vi "think_and_act.vi"(8 "error in (no error)":errorcluster, 9 "antState":T1, 10 "pieceOfWorld":T4[][](array[typedef]), 11 "Igor_1 in":refnum<class "Igor_1.lvclass">) -> (0 "error out":errorcluster, 2 "action":T2, 3 "Igor_1 out":refnum<class "Igor_1.lvclass">)   [LabVIEW 2015, in "Igor_1.lvclass"]
doc: "Ant thinks and chooses action\nCreated by Artem Shevelev\nshevelev.pro\nartem@shevelev.pro\nLabVIEW Portal: https://labviewportal.org/memberlist.php?mode=viewprofile&u=2340"
uses:
  Igor_1.lvclass
  actors/world/typedefs/worldCell_cluster.ctl
  actors/world/typedefs/markValue_cluster.ctl
  actors/world/typedefs/markValue.ctl
  actors/world/typedefs/markVolume.ctl
  actors/world/typedefs/amountOfFood.ctl
  actors/world/typedefs/anthillType_enum.ctl
  ant_base/action_cluster.ctl
  ant_base/actionType_enum.ctl
  ant_base/antState_cluster.ctl
  ant_base/ant_base.lvclass/ant_base.ctl
  ant_base/memory_limit_const.vi
  ant_base/ant_base.lvclass
  actors/world/world.lvlib
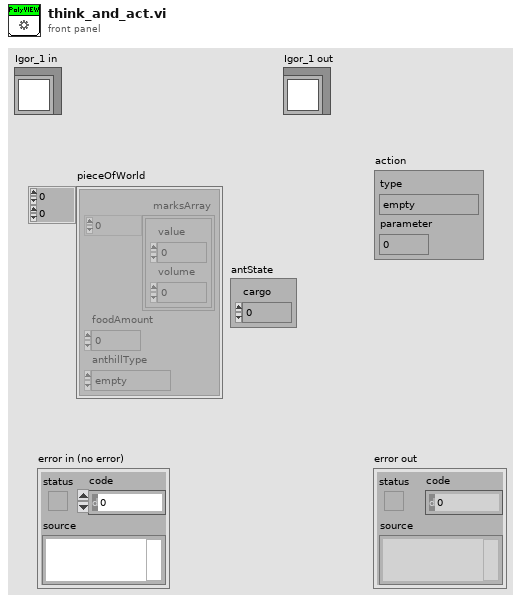
[diagram p1: front panel]
types:
  T1 = typedef "ant_base.lvclass/antState_cluster.ctl" = cluster{"cargo":u8}
  T2 = typedef "ant_base.lvclass/action_cluster.ctl" = cluster{"type":T3, "parameter":dbl}
  T3 = typedef "ant_base.lvclass/actionType_enum.ctl" = enum8{"empty", "move", "take", "put", "mark"}
  T4 = typedef "world.lvlib/worldCell_cluster.ctl" = cluster{"marksArray":T5[], "foodAmount":T8, "anthillType":T9}
  T5 = typedef "world.lvlib/markValue_cluster.ctl" = cluster{"value":T6, "volume":T7}
  T6 = typedef "world.lvlib/markValue.ctl" = u8
  T7 = typedef "world.lvlib/markVolume.ctl" = u16
  T8 = typedef "world.lvlib/amountOfFood.ctl" = i32
  T9 = typedef "world.lvlib/anthillType_enum.ctl" = enum16{"empty", "own", "rival"}
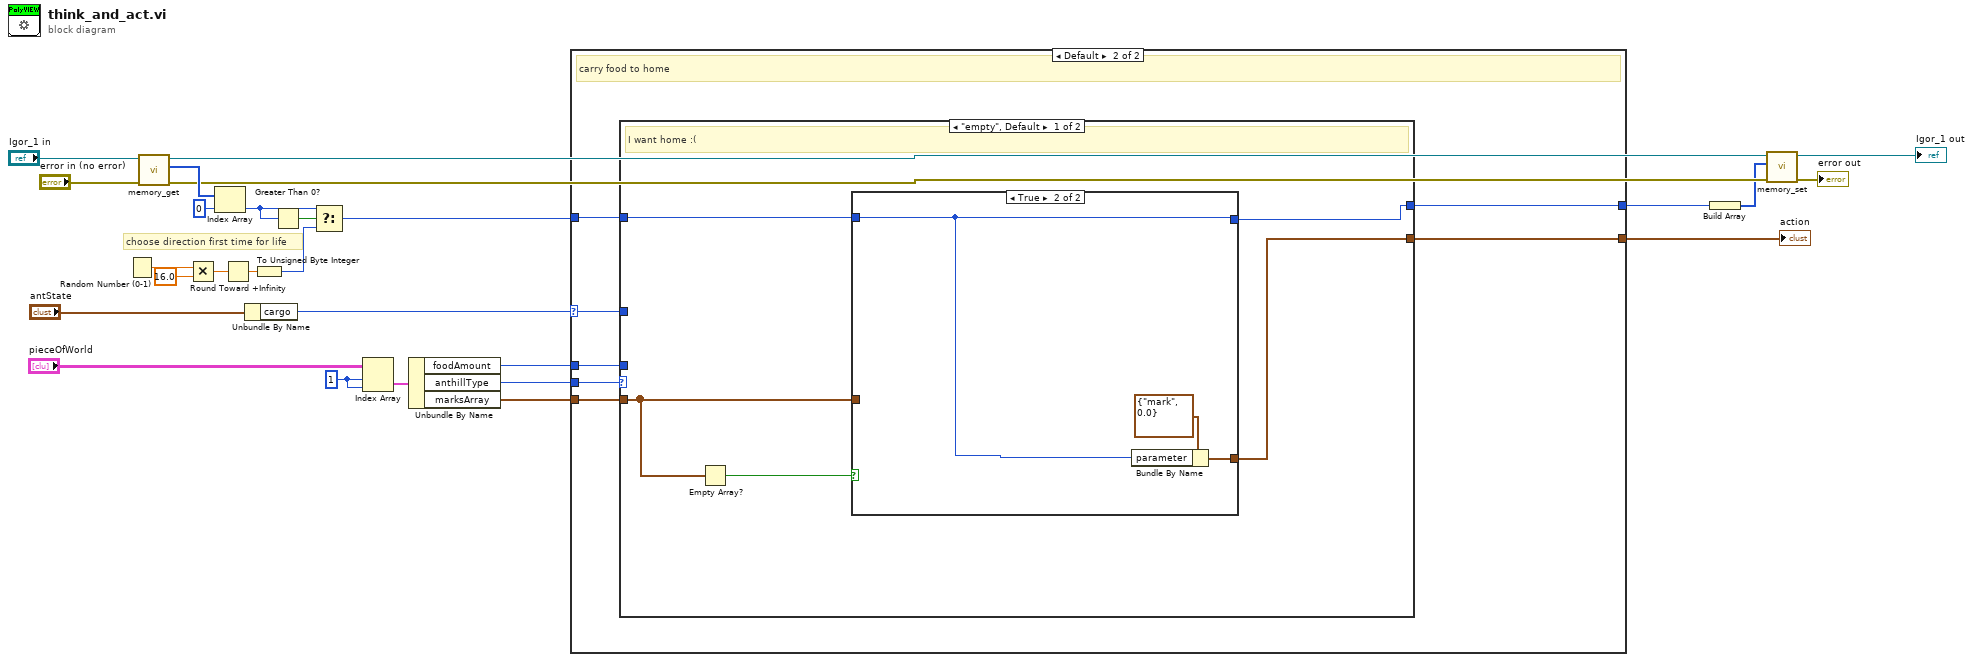
[diagram p0: block diagram]
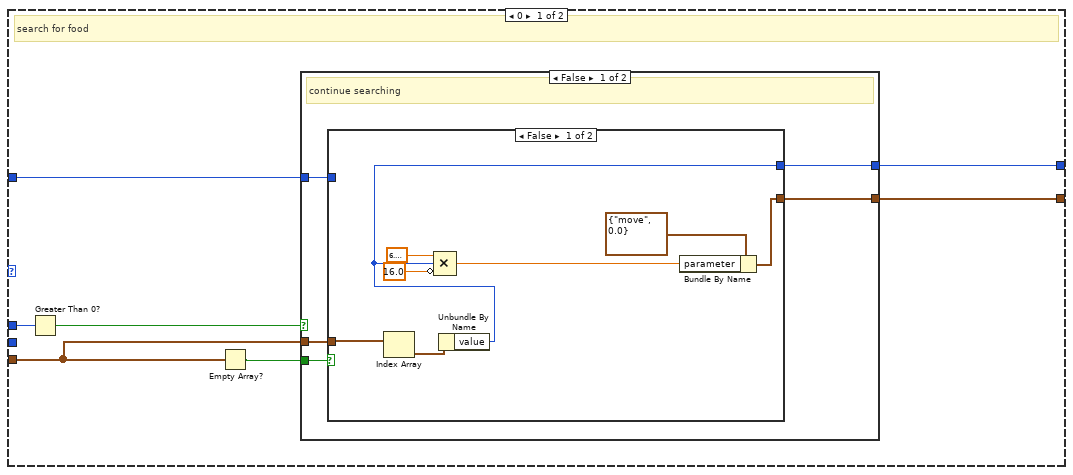
[diagram p2: hidden frame]
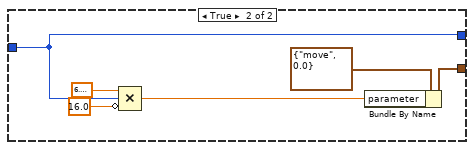
[diagram p3: hidden frame]
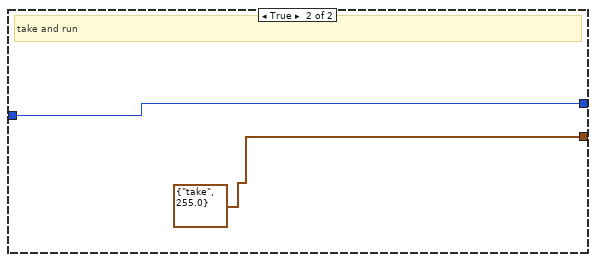
[diagram p4: hidden frame]
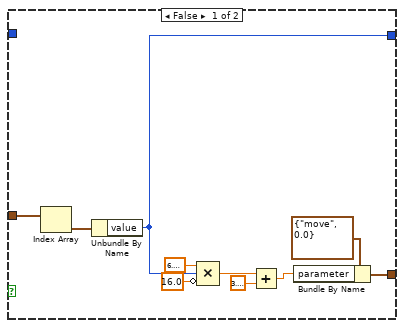
[diagram p5: hidden frame]
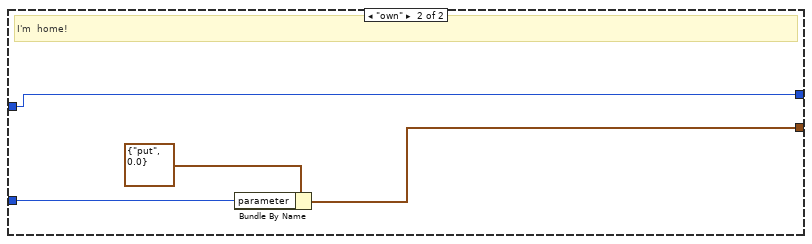
[diagram p6: hidden frame]
diagram:
  w17 = 1 ("index (row)")
  # "choose direction first time for life"
  n1 = Random Number (0-1)() -> (number: 0 to 1=w26:dbl)
  n2 = call "memory_get.vi"("error in (no error)"="error in (no error)", "ant_base in"="Igor_1 in") -> ("error out"=w18:errorcluster, "memory"=w19:u8[], "ant_base out"=w20:refnum<class "Igor_1.lvclass">)  [unwired: 7 in]
  n3 = Multiply(x=w26, y=16.0) -> (x*y=w25:dbl)
  n4 = Index Array(array=w19, index=0) -> (element=w21:u8)
  n5 = Round Toward +Infinity(x=w25) -> (ceil(x): smallest int >= x=w24:dbl)
  n6 = Unbundle By Name("antState") -> ("cargo"=w15:u8)
  n7 = To Unsigned Byte Integer(number=w24) -> (unsigned 8bit integer=w22:u8)
  n8 = Greater Than 0?(x=w21) -> (x > 0?=w23:bool)
  n9 = Select(t=w21, s=w23, f=w22) -> (s? t:f=w7:u8)
  n10 = Index Array(array="pieceOfWorld", index (row)=w17, index (col)=w17) -> (element=w16:T4)
  n11 = Unbundle By Name(w16) -> ("foodAmount"=w14:T8, "anthillType"=w13:T9, "marksArray"=w1:T5[])
  n12 = case shown="Default" w15 {
    selector: w15 -> [_ w59]
    tunnel: w14 -> [w34 w61]
    tunnel: w13 -> [_ w62]
    tunnel: [w32 w60] -> w8
    tunnel: w7 -> [w31 w58]
    tunnel: [w30 w57] -> w6
    tunnel: w1 -> [w28 w56]
    frame 0 {
      # "search for food"
      n13 = Greater Than 0?(x=w34) -> (x > 0?=w33:bool)
      n14 = Empty Array?(array=w28) -> (empty?=w29:bool)
      n15 = case shown="False" w33 {
        tunnel: [w39 T2 {"type"=enum."take", "parameter"=255.0} ("action")] -> w32
        tunnel: w31 -> [w37 w55]
        tunnel: [w38 w55] -> w30
        tunnel: w29 -> [w36 _]
        tunnel: w28 -> [w35 _]
        frame False {
          # "continue searching"
          n16 = case shown="False" w36 {
            tunnel: [w40 w52] -> w39
            tunnel: [w41 w48] -> w38
            tunnel: w37 -> [_ w48]
            tunnel: w35 -> [w47 _]
            frame False {
              n17 = Index Array(array=w47) -> (element=w42:T5)  [unwired: 1 in]
              n18 = Unbundle By Name(w42) -> ("value"=w41:T6)
              n19 = Compound Arithmetic op=MULTIPLY(6.283185307179586, w41, invert 16.0 ("y")) -> (w43:dbl)
              n20 = Bundle By Name(cluster=T2 {"type"=enum."move", "parameter"=0.0} ("action"), "parameter"=w43) -> (w40:T2)
            }
            frame True {
              n21 = Compound Arithmetic op=MULTIPLY(6.283185307179586, w48, invert 16.0 ("y")) -> (w49:dbl)
              n22 = Bundle By Name(cluster=T2 {"type"=enum."move", "parameter"=0.0} ("action"), "parameter"=w49) -> (w52:T2)
            }
          }
        }
        frame True {
          # "take and run"
        }
      }
    }
    frame Default {
      # "carry food to home"
      n23 = case shown="\"empty\", Default" w62 {
        tunnel: w61 -> [_ _]
        tunnel: [w67 w83] -> w60
        tunnel: w59 -> [_ w82]
        tunnel: w58 -> [w65 w81]
        tunnel: [w64 w81] -> w57
        tunnel: w56 -> [w63 _]
        frame "empty", Default {
          # "I want home :("
          n24 = Empty Array?(array=w63) -> (empty?=w66:bool)
          n25 = case shown="True" w66 {
            tunnel: [w76 w79] -> w67
            tunnel: w65 -> [_ w78]
            tunnel: [w68 w78] -> w64
            tunnel: w63 -> [w69 _]
            frame False {
              n26 = Index Array(array=w69) -> (element=w70:T5)  [unwired: 1 in]
              n27 = Unbundle By Name(w70) -> ("value"=w68:T6)
              n28 = Compound Arithmetic op=MULTIPLY(6.283185307179586, w68, invert 16.0 ("y")) -> (w71:dbl)
              n29 = Add(x=w71, y=3.141592653589793) -> (x+y=w75:dbl)
              n30 = Bundle By Name(cluster=T2 {"type"=enum."move", "parameter"=0.0} ("action"), "parameter"=w75) -> (w76:T2)
            }
            frame True {
              n31 = Bundle By Name(cluster=T2 {"type"=enum."mark", "parameter"=0.0} ("action"), "parameter"=w78) -> (w79:T2)
            }
          }
        }
        frame "own" {
          # "I'm  home!"
          n32 = Bundle By Name(cluster=T2 {"type"=enum."put", "parameter"=0.0} ("action"), "parameter"=w82) -> (w83:T2)
        }
      }
    }
  }
  "action" <- w8
  n33 = Build Array(w6) -> (w5:T6[])
  n34 = call "memory_set.vi"("error in (no error)"=w18, "memory"=w5, "ant_base in"=w20) -> ("error out"=→"error out":errorcluster, "ant_base out"=→"Igor_1 out":refnum<class "Igor_1.lvclass">)  [unwired: 7 in]
